vi "Ctor.vi"(8 "error in (no error)":errorcluster) -> (0 "error out":errorcluster, 3 "Callback Producer out":refnum<class "Callback Producer.lvclass">)   [LabVIEW 2020, in "Callback Producer.lvclass"]
uses:
  Callback Producer.lvclass
  Ref Data.ctl
  Callback.ctl
  Callback Producer.lvclass/Callback Producer.ctl
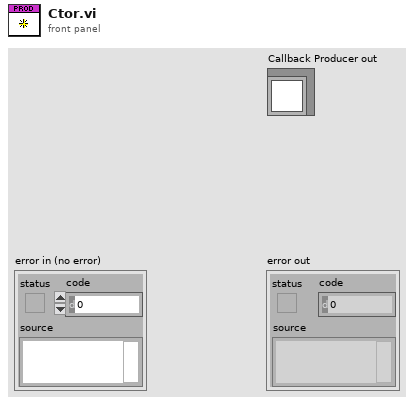
[diagram p1: front panel]
types:
  T1 = typedef "Callback Producer.lvclass/Ref Data.ctl" = cluster{"Callbacks":T2[]}
  T2 = typedef "Callback Producer.lvclass/Callback.ctl" = cluster{"Owner":refnum<class>, "VI":refnum<vi>}
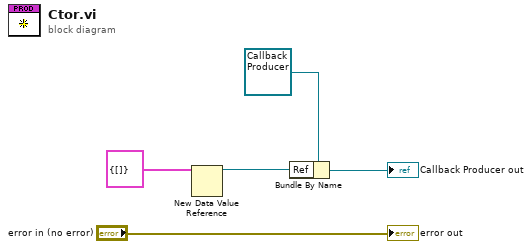
[diagram p0: block diagram]
diagram:
  n1 = New Data Value Reference(data value=T1 {"Callbacks"=[]} ("Ref Data")) -> (data value reference=w1:refnum<data-value>)  [unwired: 1 in, 1 out]
  n2 = Bundle By Name(cluster=refnum<class "Callback Producer.lvclass"> refnum ("Callback Producer in"), "Ref"=w1) -> (→"Callback Producer out":refnum<class "Callback Producer.lvclass">)
  "error out" <- "error in (no error)"
